vi "playVlc.vi"(8 "error in (no error)":errorcluster, 10 "playVlc":string, 11 "AdvancedMediaPlayer in":refnum<class "AdvancedMediaPlayer.lvclass">) -> (0 "error out":errorcluster, 3 "AdvancedMediaPlayer out":refnum<class "AdvancedMediaPlayer.lvclass">)   [LabVIEW 2018, in "AdvancedMediaPlayer.lvclass"]
uses:
  AdvancedMediaPlayer.lvclass
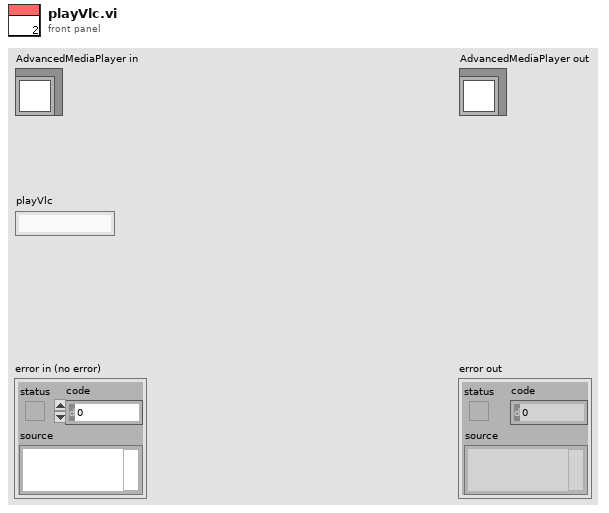
[diagram p1: front panel]
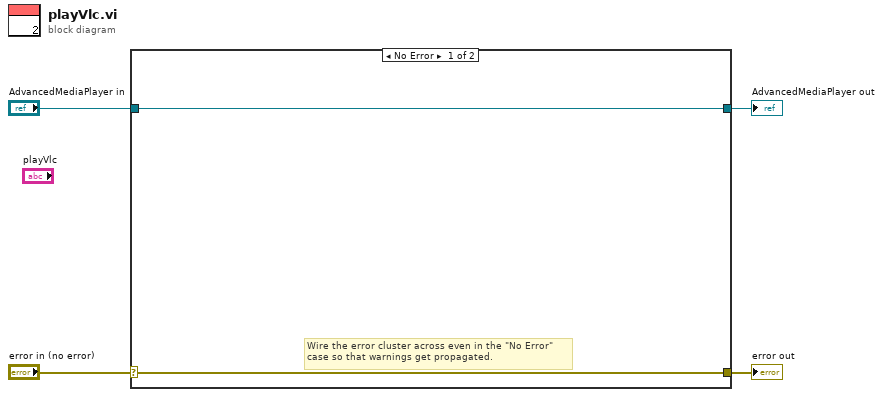
[diagram p0: block diagram]
diagram:
  n1 = case shown="No Error" "error in (no error)" {
    selector: "error in (no error)" -> [w5 w8]
    tunnel: [w5 w8] -> w3
    tunnel: [w6 w7] -> w1
    tunnel: "AdvancedMediaPlayer in" -> [w6 w7]
    frame No Error {
      # "Wire the error cluster across even in the \"No Error\"\ncase so that warnings get propagated."
    }
    frame Error {
    }
  }
  "error out" <- w3
  "AdvancedMediaPlayer out" <- w1
